vi "AngularTurn.vi"(6 "Synchronization":enum16{"Start", "Wait"}(ring), 7 "Description":string, 8 "Command Info In":T1, 10 "Speed":dbl format="%#_13g", 11 "Angle To Turn":dbl) -> (0 "Command Info Out":T1, 3 "Outcome":string="foo")   [LabVIEW 2015]
uses:
  <vilib>/Rock Robotics/WPI/Framework/Command Status Info.ctl
  <vilib>/Rock Robotics/WPI/Framework/Completion Status.ctl
  <vilib>/Rock Robotics/WPI/Framework/Completion Notifier.ctl
  Implementation/Drive Setpoints.ctl
  Implementation/Drive Operations.ctl
  NavX/NavX Global.vi
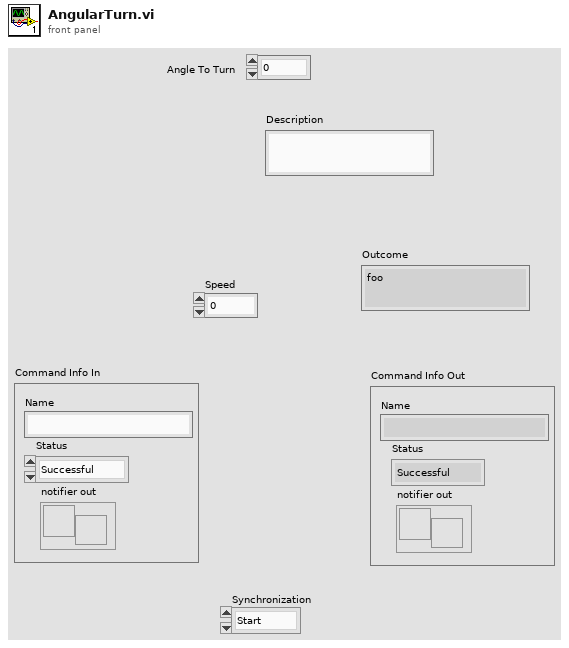
[diagram p1: front panel]
types:
  T1 = typedef "Command Status Info.ctl" = cluster{"Name":string, "Status":T2, "notifier out":T3}
  T2 = typedef "Completion Status.ctl" = enum16{"Successful", "Aborted", "Incomplete"}
  T3 = typedef "Completion Notifier.ctl" = refnum<notifier>
  T4 = typedef "Drive Setpoints.ctl" = cluster{"Operation":T5, "Left Setpoint":dbl, "Right Setpoint":dbl, "Duration":dbl, "Angle":dbl, "Distance (in)":dbl}
  T5 = typedef "Drive Operations.ctl" = enum16{"Reserve", "Read Current", "Immediate", "Drive for Time", "Drive for Distance", "Turn Degrees"}
  T6 = typedef "navX-MXP IMU.lvlib/navX YPRH Data.ctl" = cluster{"Yaw":dbl, "Pitch":dbl, "Roll":dbl, "Heading":dbl}
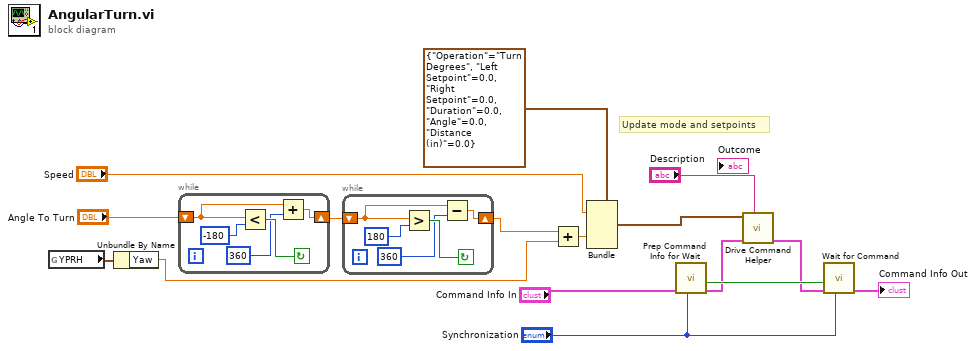
[diagram p0: block diagram]
diagram:
  # "Update mode and setpoints"
  n1 = global read "NavX Global.vi" "YPRH"() -> (w7:T6)
  n2 = Unbundle By Name(w7) -> ("Yaw"=w4:dbl)
  n3 = while {
    shift-right: [w18] -> w3
    shift-left: "Angle To Turn" -> [w20]
    stop <- w21 continue-if-true
    n4 = Less?(x=w20, y=-180) -> (x < y?=w21:bool)
    n5 = Add(x=w20, y=360) -> (x+y=w18:dbl)
  }
  n6 = while {
    shift-right: [w23] -> w2
    shift-left: w3 -> [w25]
    stop <- w26 continue-if-true
    n7 = Greater?(x=w25, y=180) -> (0:w26:bool)
    n8 = Subtract(x=w25, y=360) -> (x-y=w23:dbl)
  }
  n9 = Add(x=w2, y=w4) -> (x+y=w5:dbl)
  n10 = Bundle(cluster=T4 {"Operation"=enum."Turn Degrees", "Left Setpoint"=0.0, "Right Setpoint"=0.0, "Duration"=0.0, "Angle"=0.0, "Distance (in)"=0.0} ("SubSystem Data"), "Left Setpoint"="Speed", "Angle"=w5) -> (w9:T4)  [unwired: 4 in]
  n11 = call <vilib>:"Prep Command Info for Wait.vi"("Synchronication"="Synchronization", "Command Info"="Command Info In") -> ("Command Info"=w13:T1, "Allocated"=w14:bool)  [unwired: 8 in]
  n12 = call "Drive Command Helper.vi"("Description"="Description", "Command Info In"=w13, "SubSystem Data"=w9) -> ("Command Info Out"=w10:T1)  [unwired: 7 in, 1 out]
  n13 = call <vilib>:"Wait for Command.vi"("Synchronication"="Synchronization", "Command Info in"=w10, "Allocated"=w14) -> ("Command Info out"=→"Command Info Out":T1)  [unwired: 8 in]
